vi "Robot Main.vi"() -> ()   [LabVIEW 2025]
doc: "Robot Main serves as the primary scheduler for your command and control robotics program. It should not be necessary to modify this VI. Instead, you should add your code to the VIs called from Robot Main - Teleop, Autonomous, and SubSystems."
uses:
  <vilib>/Rock Robotics/WPI/Camera/WPI_CameraImageSize.ctl
  <vilib>/Rock Robotics/SystemInterfaces/NetworkCommunication/NetComm_UsageReport_ResourceType.ctl
  Framework/Robot Global Data.vi
panel:
  in  "Image Size":T1=enum."320x240"
  in  "Enable Vision":bool
  in  "Finish":bool
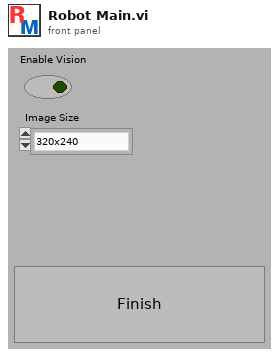
[diagram p1: front panel]
types:
  T1 = typedef "WPI_CameraImageSize.ctl" = enum16{"640x480", "320x240", "160x120", "Custom"}
  T2 = typedef "NetComm_UsageReport_ResourceType.ctl" = enum8{"Controller", "Module", "Language", "CANPlugin", "Accelerometer", "ADXL345", "AnalogChannel", "AnalogTrigger", "AnalogTriggerOutput", "CANJaguar", "Compressor", "Counter", "Dashboard", "DigitalInput", "DigitalOutput", "DriverStationCIO", "DriverStationEIO", "DriverStationLCD", "Encoder", "GearTooth", "Gyro", "I2C", "Framework", "Jaguar", "Joystick", "Kinect", "KinectStick", "PIDController", "Preferences", "PWM", "Relay", "RobotDrive", "SerialPort", "Servo", "Solenoid", "SPI", "Task", "Ultrasonic", "Victor", "Button", "Command", "AxisCamera", "PCVideoServer", "SmartDashboard", "Talon", "HiTechnicColorSensor", "HiTechnicAccel", "HiTechnicCompass", "SRF08", "AnalogOutput", "Victor SP", "Talon SRX", "CAN Talon SRX", "ADXL362 Accel", "ADXRS450 Gyro", "Rev SPARK", "Mindsensors SD540", "Digital Filter", "ADIS16448", "PDP", "PCM", "PigeonIMU", "Nidec Brushless", "CTRE CANifier", "CTRE TalonFX", "CTRE Future 1", "CTRE Future 2", "CTRE Future 3", "CTRE Future 4", "CTRE Future 5", "CTRE Future 6", "Linear Filter", "Xbox Controller", "USB Camera", "NavX", "Pixy", "Pixy2", "ScanseSweep", "Shuffleboard", "CAN", "Digilent DMC60", "PWM Victor SPX", "Rev SPARK MAX PWM", "Rev SPARK MAX CAN", "ADIS16470", "PIDController2", "ProfiledPIDController", "Kinematics", "Odometry", "Units", "Trapezoid Profile", "DutyCycle", "Addressable LEDs", "Fusion Venom", "CTRE Future 7", "CTRE Future 8", "CTRE Future 9", "CTRE Future 10", "CTRE Future 11", "CTRE Future 12", "CTRE Future 13", "CTRE Future 14", "Exponential Profile", "PS4 Controller", "Photon Camera", "Photon Pose Estimator", "Path Planner Path", "Path Planner Auto", "Path Finding Command", "Redux Future 1", "Redux Future 2", "Redux Future 3", "Redux Future 4", "Redux Future 5", "Rev SPARK Flex CAN", "Rev SPARK Flex PWM", "LEDPattern", "LinearQuadraticRegulator", "KalmanFilter", "PoseEstimator", "PoseEstimator3d", "LinearSystemLoop", "WPILib_future7", "WPILib_future8", "Rev_ServoHub", "YAMS", "LumenLabs_ConnectorX", "LumenLabs_ConnectorXLED"}
  T3 = typedef "WPI_DriverStationMatch Info.ctl" = cluster{"Autonomous Elapsed Seconds":dbl, "TeleOp Elapsed Seconds":dbl, "Disabled Elapsed Seconds":dbl, "Visited Autonomous":bool, "Visited TeleOp":bool, "Visited Disabled":bool, "Autonomous Settings":cluster{"Autonomous Style":enum16{"Iterative", "Independent"}, "VI Refnum":refnum<vi>}}
  T4 = typedef "WPI_DriverStationDerivedRobotMode.ctl" = enum16{"Init", "Execute", "Stop"}
  T5 = typedef "WPI_DriverStationRobotMode2.ctl" = enum16{"Autonomous Disabled", "Autonomous Enabled", "Teleop Disabled", "Teleop Enabled", "Disconnected", "Finish", "Test Disabled", "Test Enabled", "Emergency Stopped"}
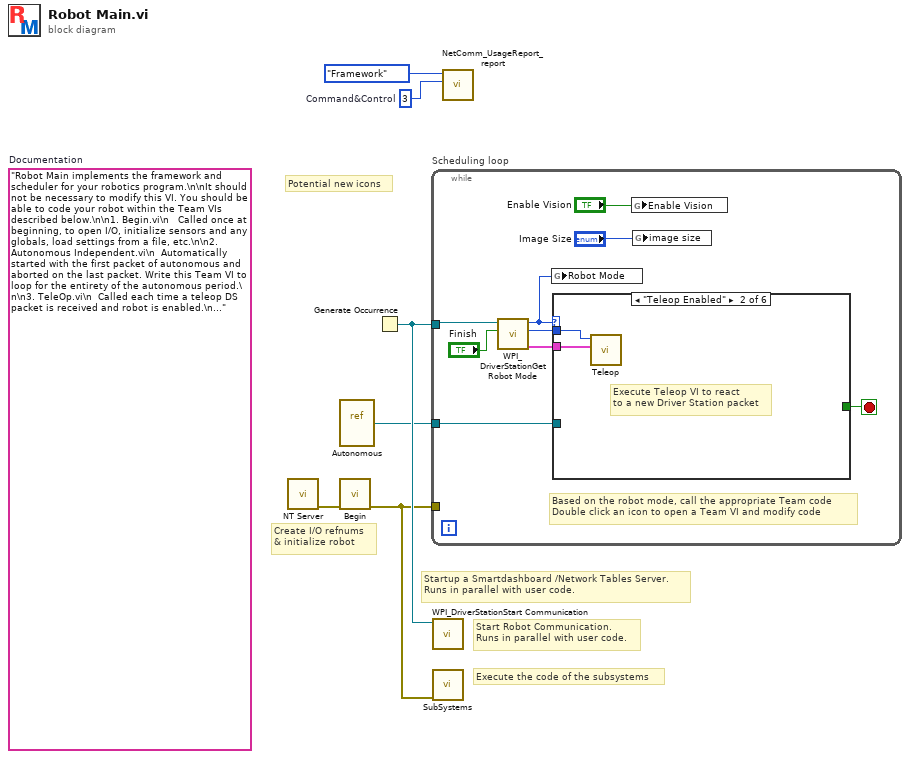
[diagram p0: block diagram]
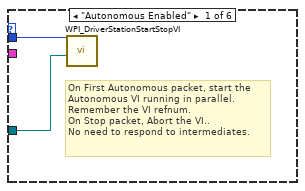
[diagram p2: hidden frame]
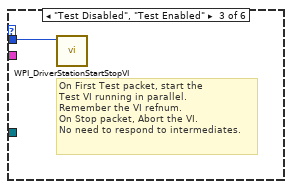
[diagram p3: hidden frame]
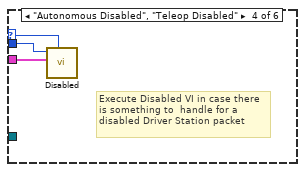
[diagram p4: hidden frame]
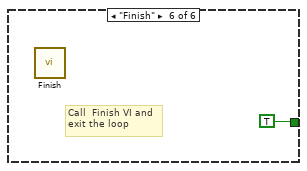
[diagram p6: hidden frame]
diagram:
  w3 = u8 3  # Command&Control
  (unwired) "Robot Main implements the framework and scheduler for your robotics program.\n\nIt should not be necessary to modify this VI. You should be able to code your robot within the Team VIs described below.\n\n1. Begin.vi\n   Called once at beginning, to open I/O, initialize sensors and any globals, load settings from a file, etc.\n\n2. Autonomous Independent.vi\n  Automatically started with the first packet of autonomous and aborted on the last packet. Write this Team VI to loop for the entirety of the autonomous period.\n\n3. TeleOp.vi\n  Called each time a teleop DS packet is received and robot is enabled.\n\n4. Disabled.vi\n  Called each time a packet is received and the robot is disabled.\n\n5. Test.vi\n  Called Automatically started with the first test packet and aborted on the last. Modify this VI to carry out robot and sensor validation tests.\n\n6. PeriodicTasks.vi\n  Parallel loops running at user-defined rates.\n\n7. Finish.vi\n  Called before exiting, so you can save data, clean up I/O, etc.\n"  # Documentation
  # "Startup a Smartdashboard /Network Tables Server.\nRuns in parallel with user code."
  # "Execute the code of the subsystems"
  # "Start Robot Communication.\nRuns in parallel with user code."
  # "Potential new icons"
  # "Create I/O refnums\n& initialize robot"
  n1 = call <vilib>:"NT Server.vi"() -> ("error out"=w2:errorcluster)  [unwired: 11 in]
  n2 = vi-ref "Autonomous.vi"() -> (w5:refnum<vi>)
  n3 = call "Begin.vi"("error in"=w2) -> ("error out"=w1:errorcluster)  [unwired: 1 in, 9 out]
  n4 = Generate Occurrence() -> (w6:refnum<k4>)
  n5 = while "Scheduling loop" {
    tunnel: w6 -> [w14]
    tunnel: w5 -> [w9]
    tunnel: w1 -> [_]
    stop <- w11 stop-if-true
    # "Based on the robot mode, call the appropriate Team code\nDouble click an icon to open a Team VI and modify code"
    n6 = call <vilib>:"WPI_DriverStationGet Robot Mode.vi"("Finish"="Finish", "DS Occurrence"=w14) -> ("Match Info out"=w12:T3, "Call Context"=w15:T4, "Robot Mode"=w7:T5)  [unwired: 7 out]
    n7 = global write "Robot Global Data.vi" "Robot Mode"(w7) -> ()
    n8 = case shown="\"Teleop Enabled\"" w7 {
      selector: w7 -> [_ _ _ w21 _ _]
      tunnel: w15 -> [w17 w19 w20 w23 _ _]
      tunnel: w12 -> [_ w18 _ w22 _ _]
      tunnel: [_ _ _ _ _ TRUE] -> w11
      tunnel: w9 -> [w16 _ _ _ _ _]
      frame "Autonomous Enabled" {
        # "On First Autonomous packet, start the\nAutonomous VI running in parallel.\nRemember the VI refnum.\nOn Stop packet, Abort the VI..\nNo need to respond to intermediates."
        n9 = call <vilib>:"WPI_DriverStationStartStopVI.vi"("VI in"=w16, "Call Context"=w17) -> ()  [unwired: 10 in]
      }
      frame "Teleop Enabled" {
        # "Execute Teleop VI to react\nto a new Driver Station packet"
        n10 = call "Teleop.vi"("Match Info"=w18, "Call Context"=w19) -> ()  [unwired: 1 in, 9 out]
      }
      frame "Test Disabled", "Test Enabled" {
        # "On First Test packet, start the\nTest VI running in parallel.\nRemember the VI refnum.\nOn Stop packet, Abort the VI.\nNo need to respond to intermediates."
        n11 = call <vilib>:"WPI_DriverStationStartStopVI.vi"("Call Context"=w20) -> ()  [unwired: 11 in]
      }
      frame "Autonomous Disabled", "Teleop Disabled" {
        # "Execute Disabled VI in case there\nis something to  handle for a\ndisabled Driver Station packet"
        n12 = call "Disabled.vi"("Robot Mode"=w21, "Match Info"=w22, "Call Context"=w23) -> ()  [unwired: 1 in, 8 out]
      }
      frame "Disconnected", Default {
        # "Driver Station packet didn't arrive.\nPossibly useful for diagnostics"
      }
      frame "Finish" {
        # "Call  Finish VI and\nexit the loop"
        n13 = call "Finish.vi"() -> ()  [unwired: 1 in, 7 out]
      }
    }
    n14 = global write "Robot Global Data.vi" "Enable Vision"("Enable Vision") -> ()
    n15 = global write "Robot Global Data.vi" "image size"("Image Size") -> ()
  }
  n16 = call <vilib>:"WPI_DriverStationStart Communication.vi"("occurrence"=w6) -> ()  [unwired: 2 in, 9 out]
  n17 = call "SubSystems.vi"("error in"=w1) -> ()  [unwired: 11 in]
  n18 = call <vilib>:"NetComm_UsageReport_report.vi"("Instance Number"=w3, "Resource Type"=NetComm_UsageReport_ResourceType."Framework") -> ()  [unwired: 10 in]
